vi "Version_2.0_Single_Column_Code.vi"() -> ()   [LabVIEW 2020] (continued)
                                n7833 = local read "Stop for End of \nExperiment \nand Data Writing"() -> (w8307:bool)
                                n7834 = call <vilib>:"Trim Whitespace.vi"("string"=w8319) -> ("trimmed string"=w8318:string)  [unwired: 1 in]
                                n7835 = Not(x=w8313) -> (.not. x?=w8311:bool)
                                n7836 = Equal?(x=w8318, y="/0`\u0003") -> (x = y?=w8316:bool)
                                n7837 = Or(x=w8311, y=w8310) -> (x .or. y?=w8309:bool)
                                n7838 = local read "Re-SEC"() -> (w8306:bool)
                                n7839 = Or(x=w8307, y=w8306) -> (x .or. y?=w8305:bool)
                                n7840 = Or(x=w8309, y=w8305) -> (x .or. y?=w8315:bool)
                                n7841 = Or(x=w8316, y=w8315) -> (x .or. y?=w8314:bool)
                                }
                                }
                                n7842 = Wait (ms)(milliseconds to wait=u32 100) -> ()  [unwired: 1 out]
                                }
                                n7843 = local write "Valve V2 Open"(FALSE ("Valve V2 Open")) -> ()
                                n7844 = local write "Valve V1 Open"(TRUE ("Valve V1 Open")) -> ()
                                n7845 = local write "External Valve \nOpen"(FALSE ("External Valve \nOpen")) -> ()
                                n7846 = local write "Volume being Injected \nin this process"(0.0) -> ()
                                }
                                frame #1 {
                                # "Keeps the on-chip valve V1, V2 and V3 closed,\nHalts also deposition onto the grid\nand waits for the 1st redeposit command. Once the command is issued\nit starts pumpoing and moves onto the next frame"
                                n7847 = stacked-sequence {
                                frame #0 {
                                n7848 = local write "Valve V1 Open"(FALSE ("Valve V1 Open")) -> ()
                                n7849 = local read "VISA Refnum in\nfor Pump"() -> (w8326:refnum<visa-resource-name>)
                                n7850 = local write "Valve V2 Open"(FALSE ("Valve V2 Open")) -> ()
                                n7851 = local write "Re-deposit Sample\nonto Grid"(FALSE ("Redeposit Sample\nonto Grid")) -> ()
                                n7852 = local write "Pause Data Collection"(TRUE ("Pause Data Collection")) -> ()
                                n7853 = call "HardStopCurrentProcess (SubVI).vi"("VISA Refnum in"=w8326) -> ()  [unwired: 11 in]
                                n7854 = local write "External Valve \nOpen"(FALSE ("External Valve \nOpen")) -> ()
                                }
                                frame #1 {
                                n7855 = while {
                                stop <- w8332 stop-if-true
                                n7856 = local read "Stop for End of \nExperiment \nand Data Writing"() -> (w8330:bool)
                                n7857 = local read "Re-SEC"() -> (w8331:bool)
                                n7858 = local read "Re-deposit Sample\nonto Grid"() -> (w8333:bool)
                                n7859 = Or(x=w8330, y=w8331) -> (x .or. y?=w8329:bool)
                                n7860 = Or(x=w8333, y=w8329) -> (x .or. y?=w8332:bool)
                                }
                                n7861 = local write "Discard fluid \nprior to 1st \ndeposition"(FALSE ("Discard fluid \nprior to 1st \ndeposition")) -> ()
                                n7862 = One Button Dialog(message="Do you want to deposit sample on another grid? If yes, turn on 'Re-deposit Sample onto Grid'. Else turn on Re-SEC to do SEC again or STOP to end the experiment") -> ()  [unwired: 1 in, 1 out]
                                }
                                frame #2 {
                                n7863 = local write "Valve V1 Open"(TRUE ("Valve V3 Open")) -> ()
                                }
                                frame #3 {
                                n7864 = local read "Re-deposit Sample\nonto Grid"() -> (w8335:bool)
                                n7865 = case shown="True" w8335 {
                                frame False {
                                n7866 = local write "Suction On/Off"(FALSE ("Suction On/Off")) -> ()
                                }
                                frame True {
                                n7867 = stacked-sequence {
                                frame #0 {
                                n7868 = local read "VISA Refnum in\nfor Pump"() -> (w8338:refnum<visa-resource-name>)
                                n7869 = call "AbsolutePlungerPosition (SubVI).vi"("VISA Refnum in"=w8338) -> ("Plunger Position"=w8337:i32)  [unwired: 10 in]
                                n7870 = local write "Position\nNow"(w8337) -> ()
                                }
                                frame #1 {
                                n7871 = local read "Buffer-B Pumping\nResolution"() -> (w8340:T2)
                                n7872 = case shown="\"Standard Pumping\", Default" w8340 {
                                tunnel: [w8341 w8352] -> w8339
                                frame "Standard Pumping", Default {
                                n7873 = local read "Buffer-B Volume \nto be  Pumped"() -> (w8344:dbl)
                                n7874 = local read "Volume of Syringe"() -> (w8347:dbl)
                                n7875 = local read "Initial Plunger Position"() -> (w8351:dbl)
                                n7876 = local read "Position\nNow"() -> (w8350:dbl)
                                n7877 = Subtract(x=w8351, y=w8350) -> (x-y=w8349:dbl)
                                n7878 = Absolute Value(x=w8349) -> (abs(x)=w8348:dbl)
                                n7879 = Multiply(x=w8348, y=w8347) -> (x*y=w8346:dbl)
                                n7880 = Divide(x=w8346, y=3000.0) -> (x/y=w8343:dbl)
                                n7881 = Subtract(x=w8343, y=w8344) -> (x-y=w8342:dbl)
                                n7882 = Absolute Value(x=w8342) -> (abs(x)=w8341:dbl)
                                }
                                frame "High Resolution Pumping" {
                                n7883 = local read "Buffer-C2 Volume \nto be Pumped"() -> (w8355:dbl)
                                n7884 = local read "Volume of Syringe"() -> (w8358:dbl)
                                n7885 = local read "Initial Plunger Position"() -> (w8362:dbl)
                                n7886 = local read "Position\nNow"() -> (w8361:dbl)
                                n7887 = Subtract(x=w8362, y=w8361) -> (x-y=w8360:dbl)
                                n7888 = Absolute Value(x=w8360) -> (abs(x)=w8359:dbl)
                                n7889 = Multiply(x=w8359, y=w8358) -> (x*y=w8357:dbl)
                                n7890 = Divide(x=w8357, y=24000.0) -> (x/y=w8354:dbl)
                                n7891 = Subtract(x=w8354, y=w8355) -> (x-y=w8353:dbl)
                                n7892 = Absolute Value(x=w8353) -> (abs(x)=w8352:dbl)
                                }
                                }
                                n7893 = local write "Buffer-C Volume\nleft to be Pumped"(w8339) -> ()
                                }
                                frame #2 {
                                n7894 = local read "Buffer-B Dispense\nFlow Rate (ul/min)"() -> (w8366:dbl)
                                n7895 = local read "Buffer-B Pumping\nResolution"() -> (w8365:T2)
                                n7896 = local read "VISA Refnum in\nfor Pump"() -> (w8368:refnum<visa-resource-name>)
                                n7897 = local read "Volume of Syringe"() -> (w8367:dbl)
                                n7898 = call "GoToAbsolutePosition(SubVI).vi"("Absolute Volume Position in Syringe (in ul)"=0.0, "Volume of Syringe"=w8367, "Resolution of Pumping"=w8365, "Flow Rate (ul/min)"=w8366, "VISA Refnum in"=w8368) -> ()  [unwired: 6 in, 1 out]
                                n7899 = local write "Suction On/Off"(FALSE ("Suction On/Off")) -> ()
                                }
                                }
                                }
                                }
                                }
                                frame #4 {
                                n7900 = local read "Stop for End of \nExperiment \nand Data Writing"() -> (w8371:bool)
                                n7901 = local read "Re-SEC"() -> (w8370:bool)
                                n7902 = Or(x=w8371, y=w8370) -> (x .or. y?=w8369:bool)
                                n7903 = case shown="True" w8369 {
                                frame False {
                                }
                                frame True {
                                n7904 = local read "VISA Refnum in\nfor Pump"() -> (w8372:refnum<visa-resource-name>)
                                n7905 = call "HardStopCurrentProcess (SubVI).vi"("VISA Refnum in"=w8372) -> ()  [unwired: 11 in]
                                }
                                }
                                }
                                }
                                }
                                frame #2 {
                                # "Keeps the on-chip valve V1, V2 Open and V3 closed"
                                n7906 = while {
                                stop <- w8378 stop-if-true
                                n7907 = local read "Suction On/Off"() -> (w8379:bool)
                                n7908 = case shown="True" w8379 {
                                frame False {
                                n7909 = local read "Initial Plunger Position"() -> (w8384:dbl)
                                n7910 = local read "Buffer-B Pumping\nResolution"() -> (w8385:T2)
                                n7911 = local read "VISA Refnum in\nfor Pump"() -> (w8386:refnum<visa-resource-name>)
                                n7912 = local read "Position\nNow"() -> (w8382:dbl)
                                n7913 = local read "Volume of Syringe"() -> (w8383:dbl)
                                n7914 = local write "Volume being Injected \nin this process"(0.0) -> ()
                                n7915 = local write "Pause Data Collection"(FALSE) -> ()
                                n7916 = while {
                                tunnel: w8386 -> [w8393]
                                tunnel: w8385 -> [w8392]
                                tunnel: w8384 -> [w8388]
                                tunnel: w8383 -> [w8391]
                                tunnel: w8382 -> [w8387]
                                stop <- w8389 stop-if-true
                                n7917 = stacked-sequence {
                                tunnel: w8393 -> [w8399 w8421 w8448]
                                tunnel: w8392 -> [w8398 w8420 _]
                                tunnel: w8388 -> [w8396 _ _]
                                tunnel: w8391 -> [w8395 w8418 _]
                                tunnel: [_ _ w8441] -> w8389
                                tunnel: w8387 -> [_ w8416 _]
                                frame #0 {
                                # "From here on 'True Volume being injected \nin this process' represents the true total \nvolume in this process"
                                n7918 = call "AbsolutePlungerPosition (SubVI).vi"("VISA Refnum in"=w8399) -> ("Plunger Position"=w8397:i32)  [unwired: 10 in]
                                n7919 = case shown="..\"Standard Pumping\"" w8398 {
                                tunnel: w8397 -> [w8407 w8415]
                                tunnel: w8396 -> [w8406 w8414]
                                tunnel: w8395 -> [w8403 w8411]
                                tunnel: [w8400 w8408] -> w8394
                                frame .."Standard Pumping" {
                                n7920 = Subtract(x=w8407, y=w8406) -> (x-y=w8405:dbl)
                                n7921 = Absolute Value(x=w8405) -> (abs(x)=w8404:dbl)
                                n7922 = Multiply(x=w8404, y=w8403) -> (x*y=w8402:dbl)
                                n7923 = Divide(x=w8402, y=3000.0) -> (x/y=w8400:dbl)
                                }
                                frame "High Resolution Pumping".. {
                                n7924 = Subtract(x=w8415, y=w8414) -> (x-y=w8413:dbl)
                                n7925 = Absolute Value(x=w8413) -> (abs(x)=w8412:dbl)
                                n7926 = Multiply(x=w8412, y=w8411) -> (x*y=w8410:dbl)
                                n7927 = Divide(x=w8410, y=24000.0) -> (x/y=w8408:dbl)
                                }
                                }
                                n7928 = local write "True Volume being \ninjected in this\nprocess"(w8394) -> ()
                                }
                                frame #1 {
                                # "From here on 'Volume being injected \nin this process' represents the volume \nin this sub process"
                                n7929 = call "AbsolutePlungerPosition (SubVI).vi"("VISA Refnum in"=w8421) -> ("Plunger Position"=w8419:i32)  [unwired: 10 in]
                                n7930 = case shown="\"High Resolution Pumping\".." w8420 {
                                tunnel: w8419 -> [w8429 w8437]
                                tunnel: w8416 -> [w8428 w8436]
                                tunnel: w8418 -> [w8425 w8433]
                                tunnel: [w8422 w8430] -> w8417
                                frame .."Standard Pumping" {
                                n7931 = Subtract(x=w8429, y=w8428) -> (x-y=w8427:dbl)
                                n7932 = Absolute Value(x=w8427) -> (abs(x)=w8426:dbl)
                                n7933 = Multiply(x=w8426, y=w8425) -> (x*y=w8424:dbl)
                                n7934 = Divide(x=w8424, y=3000.0) -> (x/y=w8422:dbl)
                                }
                                frame "High Resolution Pumping".. {
                                n7935 = Subtract(x=w8437, y=w8436) -> (x-y=w8435:dbl)
                                n7936 = Absolute Value(x=w8435) -> (abs(x)=w8434:dbl)
                                n7937 = Multiply(x=w8434, y=w8433) -> (x*y=w8432:dbl)
                                n7938 = Divide(x=w8432, y=24000.0) -> (x/y=w8430:dbl)
                                }
                                }
                                n7939 = local write "Volume being Injected \nin this process"(w8417) -> ()
                                }
                                frame #2 {
                                n7940 = local read "Stop for End of \nExperiment \nand Data Writing"() -> (w8440:bool)
                                n7941 = local read "Re-SEC"() -> (w8439:bool)
                                n7942 = local read "Suction On/Off"() -> (w8444:bool)
                                n7943 = call "AbsolutePlungerPositionStatus (SubVI).vi"("VISA Refnum in"=w8448) -> ("read buffer"=w8447:string)  [unwired: 10 in]
                                n7944 = call <vilib>:"Trim Whitespace.vi"("string"=w8447) -> ("trimmed string"=w8446:string)  [unwired: 1 in]
                                n7945 = Equal?(x=w8446, y="/0`\u0003") -> (x = y?=w8443:bool)
                                n7946 = Or(x=w8440, y=w8439) -> (x .or. y?=w8438:bool)
                                n7947 = Or(x=w8444, y=w8438) -> (x .or. y?=w8442:bool)
                                n7948 = Or(x=w8443, y=w8442) -> (x .or. y?=w8441:bool)
                                }
                                }
                                n7949 = Wait (ms)(milliseconds to wait=u32 100) -> ()  [unwired: 1 out]
                                }
                                }
                                frame True {
                                n7950 = stacked-sequence {
                                frame #0 {
                                n7951 = local write "Valve V1 Open"(FALSE ("Valve V3 Open")) -> ()
                                n7952 = local read "Suction Pressure\nfor EM-grid \nDeposition (mbar)"() -> (w8450:sgl)
                                n7953 = local read "VISA Refnum in\nfor Pump"() -> (w8453:refnum<visa-resource-name>)
                                n7954 = local write "Suction pressure \nfor grid deposition"(w8450) -> ()
                                n7955 = local write "Re-deposit Sample\nonto Grid"(FALSE ("Redeposit Sample\nonto Grid")) -> ()
                                n7956 = local write "Pause Data Collection"(TRUE ("Pause Data Collection")) -> ()
                                n7957 = call "HardStopCurrentProcess (SubVI).vi"("VISA Refnum in"=w8453) -> ()  [unwired: 11 in]
                                }
                                frame #1 {
                                n7958 = while {
                                stop <- w8456 stop-if-true
                                n7959 = local read "Stop for End of \nExperiment \nand Data Writing"() -> (w8457:bool)
                                n7960 = local read "Suction Pressure\nfor EM-grid \nDeposition (mbar)"() -> (w8454:sgl)
                                n7961 = call <vilib>:"fgt set pressure.vi"("pressure"=w8454, "pressureIndex"=u32 1) -> ()  [unwired: 9 in, 1 out]
                                n7962 = local read "Suction On/Off"() -> (w8459:bool)
                                n7963 = Not(x=w8459) -> (.not. x?=w8458:bool)
                                n7964 = Wait (ms)(milliseconds to wait=u32 100) -> ()  [unwired: 1 out]
                                n7965 = Or(x=w8458, y=w8457) -> (x .or. y?=w8456:bool)
                                }
                                }
                                frame #2 {
                                n7966 = for {
                                N: 2 -> [_]
                                n7967 = while {
                                stop <- w8469 stop-if-true
                                n7968 = local read "Stop for End of \nExperiment \nand Data Writing"() -> (w8465:bool)
                                n7969 = local read "Suction On/Off"() -> (w8467:bool)
                                n7970 = call <vilib>:"fgt set pressure.vi"("pressure"=sgl 0.0, "pressureIndex"=u32 1) -> ()  [unwired: 9 in, 1 out]
                                n7971 = Not(x=w8467) -> (.not. x?=w8466:bool)
                                n7972 = Wait (ms)(milliseconds to wait=u32 100) -> ()  [unwired: 1 out]
                                n7973 = Or(x=w8466, y=w8465) -> (x .or. y?=w8469:bool)
                                }
                                n7974 = Wait (ms)(milliseconds to wait=u32 400) -> ()  [unwired: 1 out]
                                }
                                }
                                frame #3 {
                                n7975 = local read "Automatic purging \nof capillary after \ngrid deposition"() -> (w8470:bool)
                                n7976 = case shown="True" w8470 {
                                frame False {
                                }
                                frame True {
                                n7977 = stacked-sequence {
                                frame #0 {
                                n7978 = local read "VISA Refnum in\nfor Pump"() -> (w8472:refnum<visa-resource-name>)
                                n7979 = call "AbsolutePlungerPosition (SubVI).vi"("VISA Refnum in"=w8472) -> ("Plunger Position"=w8471:i32)  [unwired: 10 in]
                                n7980 = local write "Position\nNow"(w8471) -> ()
                                }
                                frame #1 {
                                n7981 = local read "Buffer-B Pumping\nResolution"() -> (w8474:T2)
                                n7982 = case shown="\"Standard Pumping\", Default" w8474 {
                                tunnel: [w8475 w8486] -> w8473
                                frame "Standard Pumping", Default {
                                n7983 = local read "Buffer-B Volume \nto be  Pumped"() -> (w8478:dbl)
                                n7984 = local read "Volume of Syringe"() -> (w8481:dbl)
                                n7985 = local read "Initial Plunger Position"() -> (w8485:dbl)
                                n7986 = local read "Position\nNow"() -> (w8484:dbl)
                                n7987 = Subtract(x=w8485, y=w8484) -> (x-y=w8483:dbl)
                                n7988 = Absolute Value(x=w8483) -> (abs(x)=w8482:dbl)
                                n7989 = Multiply(x=w8482, y=w8481) -> (x*y=w8480:dbl)
                                n7990 = Divide(x=w8480, y=3000.0) -> (x/y=w8477:dbl)
                                n7991 = Subtract(x=w8477, y=w8478) -> (x-y=w8476:dbl)
                                n7992 = Absolute Value(x=w8476) -> (abs(x)=w8475:dbl)
                                }
                                frame "High Resolution Pumping" {
                                n7993 = local read "Buffer-C2 Volume \nto be Pumped"() -> (w8489:dbl)
                                n7994 = local read "Volume of Syringe"() -> (w8492:dbl)
                                n7995 = local read "Initial Plunger Position"() -> (w8496:dbl)
                                n7996 = local read "Position\nNow"() -> (w8495:dbl)
                                n7997 = Subtract(x=w8496, y=w8495) -> (x-y=w8494:dbl)
                                n7998 = Absolute Value(x=w8494) -> (abs(x)=w8493:dbl)
                                n7999 = Multiply(x=w8493, y=w8492) -> (x*y=w8491:dbl)
                                n8000 = Divide(x=w8491, y=24000.0) -> (x/y=w8488:dbl)
                                n8001 = Subtract(x=w8488, y=w8489) -> (x-y=w8487:dbl)
                                n8002 = Absolute Value(x=w8487) -> (abs(x)=w8486:dbl)
                                }
                                }
                                n8003 = local write "Buffer-C Volume\nleft to be Pumped"(w8473) -> ()
                                }
                                frame #2 {
                                n8004 = local read "Buffer-B Dispense\nFlow Rate (ul/min)"() -> (w8500:dbl)
                                n8005 = local read "Buffer-B Pumping\nResolution"() -> (w8499:T2)
                                n8006 = local read "VISA Refnum in\nfor Pump"() -> (w8502:refnum<visa-resource-name>)
                                n8007 = local read "Volume of Syringe"() -> (w8501:dbl)
                                n8008 = call "GoToAbsolutePosition(SubVI).vi"("Absolute Volume Position in Syringe (in ul)"=0.0, "Volume of Syringe"=w8501, "Resolution of Pumping"=w8499, "Flow Rate (ul/min)"=w8500, "VISA Refnum in"=w8502) -> ()  [unwired: 6 in, 1 out]
                                n8009 = local write "Valve V1 Open"(TRUE ("Valve V3 Open")) -> ()
                                }
                                frame #3 {
                                n8010 = local read "Initial Plunger Position"() -> (w8507:dbl)
                                n8011 = local read "Buffer-B Pumping\nResolution"() -> (w8508:T2)
                                n8012 = local read "VISA Refnum in\nfor Pump"() -> (w8509:refnum<visa-resource-name>)
                                n8013 = local read "Position\nNow"() -> (w8505:dbl)
                                n8014 = local read "Volume of Syringe"() -> (w8506:dbl)
                                n8015 = local write "Volume being Injected \nin this process"(0.0) -> ()
                                n8016 = local write "Pause Data Collection"(FALSE) -> ()
                                n8017 = while {
                                tunnel: w8509 -> [w8516]
                                tunnel: w8508 -> [w8515]
                                tunnel: w8507 -> [w8511]
                                tunnel: w8506 -> [w8514]
                                tunnel: w8505 -> [w8510]
                                stop <- w8512 stop-if-true
                                n8018 = stacked-sequence {
                                tunnel: w8516 -> [w8522 w8544 w8573]
                                tunnel: w8515 -> [w8521 w8543 _]
                                tunnel: w8511 -> [w8519 _ _]
                                tunnel: w8514 -> [w8518 w8541 _]
                                tunnel: [_ _ w8567] -> w8512
                                tunnel: w8510 -> [_ w8539 _]
                                frame #0 {
                                # "From here on 'True Volume being injected \nin this process' represents the true total \nvolume in this process"
                                n8019 = call "AbsolutePlungerPosition (SubVI).vi"("VISA Refnum in"=w8522) -> ("Plunger Position"=w8520:i32)  [unwired: 10 in]
                                n8020 = case shown="..\"Standard Pumping\"" w8521 {
                                tunnel: w8520 -> [w8530 w8538]
                                tunnel: w8519 -> [w8529 w8537]
                                tunnel: w8518 -> [w8526 w8534]
                                tunnel: [w8523 w8531] -> w8517
                                frame .."Standard Pumping" {
                                n8021 = Subtract(x=w8530, y=w8529) -> (x-y=w8528:dbl)
                                n8022 = Absolute Value(x=w8528) -> (abs(x)=w8527:dbl)
                                n8023 = Multiply(x=w8527, y=w8526) -> (x*y=w8525:dbl)
                                n8024 = Divide(x=w8525, y=3000.0) -> (x/y=w8523:dbl)
                                }
                                frame "High Resolution Pumping".. {
                                n8025 = Subtract(x=w8538, y=w8537) -> (x-y=w8536:dbl)
                                n8026 = Absolute Value(x=w8536) -> (abs(x)=w8535:dbl)
                                n8027 = Multiply(x=w8535, y=w8534) -> (x*y=w8533:dbl)
                                n8028 = Divide(x=w8533, y=24000.0) -> (x/y=w8531:dbl)
                                }
                                }
                                n8029 = local write "True Volume being \ninjected in this\nprocess"(w8517) -> ()
                                }
                                frame #1 {
                                # "From here on 'Volume being injected \nin this process' represents the volume \nin this sub process"
                                n8030 = call "AbsolutePlungerPosition (SubVI).vi"("VISA Refnum in"=w8544) -> ("Plunger Position"=w8542:i32)  [unwired: 10 in]
                                n8031 = case shown="\"High Resolution Pumping\".." w8543 {
                                tunnel: w8542 -> [w8552 w8560]
                                tunnel: w8539 -> [w8551 w8559]
                                tunnel: w8541 -> [w8548 w8556]
                                tunnel: [w8545 w8553] -> w8540
                                frame .."Standard Pumping" {
                                n8032 = Subtract(x=w8552, y=w8551) -> (x-y=w8550:dbl)
                                n8033 = Absolute Value(x=w8550) -> (abs(x)=w8549:dbl)
                                n8034 = Multiply(x=w8549, y=w8548) -> (x*y=w8547:dbl)
                                n8035 = Divide(x=w8547, y=3000.0) -> (x/y=w8545:dbl)
                                }
                                frame "High Resolution Pumping".. {
                                n8036 = Subtract(x=w8560, y=w8559) -> (x-y=w8558:dbl)
                                n8037 = Absolute Value(x=w8558) -> (abs(x)=w8557:dbl)
                                n8038 = Multiply(x=w8557, y=w8556) -> (x*y=w8555:dbl)
                                n8039 = Divide(x=w8555, y=24000.0) -> (x/y=w8553:dbl)
                                }
                                }
                                n8040 = local write "Volume being Injected \nin this process"(w8540) -> ()
                                }
                                frame #2 {
                                n8041 = local read "Capillary purge \nvolume after every\ngrid plunging"() -> (w8562:dbl)
                                n8042 = local read "Stop for End of \nExperiment \nand Data Writing"() -> (w8566:bool)
                                n8043 = local read "Volume being Injected \nin this process"() -> (w8563:dbl)
                                n8044 = local read "Re-SEC"() -> (w8565:bool)
                                n8045 = call "AbsolutePlungerPositionStatus (SubVI).vi"("VISA Refnum in"=w8573) -> ("read buffer"=w8572:string)  [unwired: 10 in]
                                n8046 = call <vilib>:"Trim Whitespace.vi"("string"=w8572) -> ("trimmed string"=w8571:string)  [unwired: 1 in]
                                n8047 = Greater Or Equal?(x=w8563, y=w8562) -> (x >= y?=w8561:bool)
                                n8048 = Equal?(x=w8571, y="/0`\u0003") -> (x = y?=w8569:bool)
                                n8049 = Or(x=w8566, y=w8565) -> (x .or. y?=w8564:bool)
                                n8050 = Or(x=w8561, y=w8564) -> (x .or. y?=w8568:bool)
                                n8051 = Or(x=w8569, y=w8568) -> (x .or. y?=w8567:bool)
                                }
                                }
                                n8052 = Wait (ms)(milliseconds to wait=u32 100) -> ()  [unwired: 1 out]
                                }
                                }
                                frame #4 {
                                n8053 = local read "VISA Refnum in\nfor Pump"() -> (w8574:refnum<visa-resource-name>)
                                n8054 = call "HardStopCurrentProcess (SubVI).vi"("VISA Refnum in"=w8574) -> ()  [unwired: 11 in]
                                }
                                }
                                }
                                }
                                }
                                frame #4 {
                                n8055 = local write "Valve V1 Open"(FALSE ("Valve V3 Open")) -> ()
                                }
                                frame #5 {
                                n8056 = while {
                                stop <- w8580 stop-if-true
                                n8057 = local read "Stop for End of \nExperiment \nand Data Writing"() -> (w8578:bool)
                                n8058 = local read "Re-deposit Sample\nonto Grid"() -> (w8581:bool)
                                n8059 = local read "Re-SEC"() -> (w8579:bool)
                                n8060 = Or(x=w8578, y=w8579) -> (x .or. y?=w8577:bool)
                                n8061 = Or(x=w8581, y=w8577) -> (x .or. y?=w8580:bool)
                                }
                                n8062 = One Button Dialog(message="Do you want to deposit sample on another grid? If yes, turn on 'Re-deposit Sample onto Grid'. Else turn on Re-SEC to do SEC again or STOP to end the experiment") -> ()  [unwired: 1 in, 1 out]
                                }
                                frame #6 {
                                n8063 = local write "Valve V1 Open"(TRUE ("Valve V3 Open")) -> ()
                                }
                                frame #7 {
                                n8064 = local read "Re-deposit Sample\nonto Grid"() -> (w8583:bool)
                                n8065 = case shown="True" w8583 {
                                frame False {
                                n8066 = local write "Suction On/Off"(FALSE ("Suction On/Off")) -> ()
                                }
                                frame True {
                                n8067 = stacked-sequence {
                                frame #0 {
                                n8068 = local read "VISA Refnum in\nfor Pump"() -> (w8586:refnum<visa-resource-name>)
                                n8069 = call "AbsolutePlungerPosition (SubVI).vi"("VISA Refnum in"=w8586) -> ("Plunger Position"=w8585:i32)  [unwired: 10 in]
                                n8070 = local write "Position\nNow"(w8585) -> ()
                                }
                                frame #1 {
                                n8071 = local read "Buffer-B Pumping\nResolution"() -> (w8588:T2)
                                n8072 = case shown="\"Standard Pumping\", Default" w8588 {
                                tunnel: [w8589 w8600] -> w8587
                                frame "Standard Pumping", Default {
                                n8073 = local read "Buffer-B Volume \nto be  Pumped"() -> (w8592:dbl)
                                n8074 = local read "Volume of Syringe"() -> (w8595:dbl)
                                n8075 = local read "Initial Plunger Position"() -> (w8599:dbl)
                                n8076 = local read "Position\nNow"() -> (w8598:dbl)
                                n8077 = Subtract(x=w8599, y=w8598) -> (x-y=w8597:dbl)
                                n8078 = Absolute Value(x=w8597) -> (abs(x)=w8596:dbl)
                                n8079 = Multiply(x=w8596, y=w8595) -> (x*y=w8594:dbl)
                                n8080 = Divide(x=w8594, y=3000.0) -> (x/y=w8591:dbl)
                                n8081 = Subtract(x=w8591, y=w8592) -> (x-y=w8590:dbl)
                                n8082 = Absolute Value(x=w8590) -> (abs(x)=w8589:dbl)
                                }
                                frame "High Resolution Pumping" {
                                n8083 = local read "Buffer-C2 Volume \nto be Pumped"() -> (w8603:dbl)
                                n8084 = local read "Volume of Syringe"() -> (w8606:dbl)
                                n8085 = local read "Initial Plunger Position"() -> (w8610:dbl)
                                n8086 = local read "Position\nNow"() -> (w8609:dbl)
                                n8087 = Subtract(x=w8610, y=w8609) -> (x-y=w8608:dbl)
                                n8088 = Absolute Value(x=w8608) -> (abs(x)=w8607:dbl)
                                n8089 = Multiply(x=w8607, y=w8606) -> (x*y=w8605:dbl)
                                n8090 = Divide(x=w8605, y=24000.0) -> (x/y=w8602:dbl)
                                n8091 = Subtract(x=w8602, y=w8603) -> (x-y=w8601:dbl)
                                n8092 = Absolute Value(x=w8601) -> (abs(x)=w8600:dbl)
                                }
                                }
                                n8093 = local write "Buffer-C Volume\nleft to be Pumped"(w8587) -> ()
                                }
                                frame #2 {
                                n8094 = local read "Buffer-B Dispense\nFlow Rate (ul/min)"() -> (w8614:dbl)
                                n8095 = local read "Buffer-B Pumping\nResolution"() -> (w8613:T2)
                                n8096 = local read "VISA Refnum in\nfor Pump"() -> (w8616:refnum<visa-resource-name>)
                                n8097 = local read "Volume of Syringe"() -> (w8615:dbl)
                                n8098 = call "GoToAbsolutePosition(SubVI).vi"("Absolute Volume Position in Syringe (in ul)"=0.0, "Volume of Syringe"=w8615, "Resolution of Pumping"=w8613, "Flow Rate (ul/min)"=w8614, "VISA Refnum in"=w8616) -> ()  [unwired: 6 in, 1 out]
                                n8099 = local write "Suction On/Off"(FALSE ("Suction On/Off")) -> ()
                                }
                                }
                                }
                                }
                                }
                                frame #8 {
                                n8100 = local read "Stop for End of \nExperiment \nand Data Writing"() -> (w8618:bool)
                                n8101 = local read "Re-SEC"() -> (w8619:bool)
                                n8102 = Or(x=w8618, y=w8619) -> (x .or. y?=w8617:bool)
                                n8103 = case shown="True" w8617 {
                                frame False {
                                }
                                frame True {
                                n8104 = local read "VISA Refnum in\nfor Pump"() -> (w8620:refnum<visa-resource-name>)
                                n8105 = call "HardStopCurrentProcess (SubVI).vi"("VISA Refnum in"=w8620) -> ()  [unwired: 11 in]
                                }
                                }
                                }
                                }
                                }
                                }
                                n8106 = local read "Stop for End of \nExperiment \nand Data Writing"() -> (w8374:bool)
                                n8107 = local read "Divert Sample \nonto Grid"() -> (w8377:bool)
                                n8108 = local read "Re-SEC"() -> (w8375:bool)
                                n8109 = Not(x=w8377) -> (.not. x?=w8376:bool)
                                n8110 = Or(x=w8374, y=w8375) -> (x .or. y?=w8373:bool)
                                n8111 = Or(x=w8376, y=w8373) -> (x .or. y?=w8378:bool)
                                }
                                }
                                }
                                n8112 = local write "Discard fluid \nprior to 1st \ndeposition"(TRUE ("Discard fluid \nprior to 1st \ndeposition")) -> ()
                                }
                                }
                              }
                              frame #9 {
                                n8113 = local write "Pause Data Collection"(TRUE ("Pause Data Collection")) -> ()
                                n8114 = Wait (ms)(milliseconds to wait=u32 500) -> ()  [unwired: 1 out]
                              }
                              frame #10 {
                                n8115 = local write "Volume being Injected \nin this process"(0.0 ("Volume being Injected \nin this process")) -> ()
                                n8116 = local write "Affinity Elution On"(FALSE ("Affinity Elution On")) -> ()
                                n8117 = local write "Start the Process"(FALSE ("Start the Process")) -> ()
                              }
                            }
                          }
                        }
                        n8118 = local write "Washing Column-1"(FALSE ("Sample pumping \ninto Column-1")) -> ()
                        n8119 = local write "Elution of Column-1"(TRUE ("Washing Column-1")) -> ()
                        n8120 = local write "Affinity Elution On"(TRUE ("Affinity Elution On")) -> ()
                      }
                    }
                  }
                }
              }
              frame True {
                n8121 = local write "Pause Data Collection"(FALSE ("Pause Data Collection")) -> ()
              }
            }
          }
          frame "Inject Buffer A2, Column 1 with 4 SOD Valves" {
            n8122 = local read "Stopper that ends \nthe main loops"() -> (w8627:bool)
            n8123 = case shown="False" w8627 {
              frame False {
                n8124 = local read "Start the Process"() -> (w8628:bool)
                n8125 = case shown="True" w8628 {
                  frame False {
                    n8126 = local read "Stopper that ends \nthe main loops"() -> (w8630:bool)
                    n8127 = local read "Start the Process"() -> (w8629:bool)
                    n8128 = Or(x=w8630, y=w8629) -> (x .or. y?=w8631:bool)
                    n8129 = case shown="False" w8631 {
                      frame False {
                        n8130 = while {
                          stop <- w8634 stop-if-true
                          n8131 = local read "Stop for End of \nExperiment \nand Data Writing"() -> (w8633:bool)
                          n8132 = local read "Stopper that ends \nthe main loops"() -> (w8636:bool)
                          n8133 = local read "Start the Process"() -> (w8635:bool)
                          n8134 = Wait (ms)(milliseconds to wait=u32 10) -> ()  [unwired: 1 out]
                          n8135 = Or(x=w8636, y=w8635) -> (x .or. y?=w8634:bool)
                          n8136 = local write "Stopper that ends \nthe main loops"(w8633) -> ()
                        }
                        n8137 = One Button Dialog(message="Please Select the Process and Press 'Start the Process' Button") -> ()  [unwired: 1 in, 1 out]
                      }
                      frame True {
                      }
                    }
                  }
                  frame True {
                    n8138 = stacked-sequence {
                      frame #0 {
                        n8139 = local read "Buffer-A2 Volume \nto be Pumped"() -> (w8641:dbl)
                        n8140 = local read "Apparent Volume\nof Syringe"() -> (w8640:dbl)
                        n8141 = Quotient & Remainder(x=w8641, y=w8640) -> (x-y*floor(x/y)=w8638:dbl, floor(x/y)=w8639:dbl)
                        n8142 = for {
                          N: w8639 -> [_]
                          n8143 = stacked-sequence {
                            frame #0 {
                              # "Switch to Port-4"
                              # "Port-4 of pump is connected to Buffer-A"
                              n8144 = local read "VISA Refnum in\nfor Pump"() -> (w8643:refnum<visa-resource-name>)
                              n8145 = local read "Port for \nA2-Wash"() -> (w8642:string)
                              n8146 = call "PortChanger (SubVI).vi"("Port Number"=w8642, "VISA Refnum in"=w8643) -> ()  [unwired: 10 in]
                            }
                            frame #1 {
                              n8147 = local read "VISA Refnum in\nfor Pump"() -> (w8644:refnum<visa-resource-name>)
                              n8148 = call "ProcessCompletionWaiter (SubVI).vi"("VISA Refnum in"=w8644) -> ()  [unwired: 11 in]
                            }
                            frame #2 {
                              n8149 = local read "Buffer-A2 PickUp \nFlow Rate (ul/min)"() -> (w8647:dbl)
                              n8150 = local read "Buffer-A2 Pumping\nResolution"() -> (w8646:T2)
                              n8151 = local read "VISA Refnum in\nfor Pump"() -> (w8649:refnum<visa-resource-name>)
                              n8152 = local read "Apparent Volume\nof Syringe"() -> (w8645:dbl)
                              n8153 = local read "Volume of Syringe"() -> (w8648:dbl)
                              n8154 = call "RPickUp(SubVI).vi"("Volume to be picked up"=w8645, "Volume of Syringe"=w8648, "Resolution of PickUP"=w8646, "PickUp Flow Rate (ul/min)"=w8647, "VISA Refnum in"=w8649) -> ()  [unwired: 6 in, 1 out]
                            }
                            frame #3 {
                              n8155 = local read "Stopper that ends \nthe main loops"() -> (w8650:bool)
                              n8156 = local read "VISA Refnum in\nfor Pump"() -> (w8651:refnum<visa-resource-name>)
                              n8157 = case shown="True" w8650 {
                                frame False {
                                }
                                frame True {
                                n8158 = local read "VISA Refnum in\nfor Pump"() -> (w8652:refnum<visa-resource-name>)
                                n8159 = call "HardStopCurrentProcess (SubVI).vi"("VISA Refnum in"=w8652) -> ()  [unwired: 11 in]
                                }
                              }
                              n8160 = call "ProcessCompletionWaiter (SubVI).vi"("VISA Refnum in"=w8651) -> ()  [unwired: 11 in]
                            }
                            frame #4 {
                              # "Reads the initial Plunger Position for computing the volume dispensed"
                              n8161 = local read "VISA Refnum in\nfor Pump"() -> (w8654:refnum<visa-resource-name>)
                              n8162 = call "AbsolutePlungerPosition (SubVI).vi"("VISA Refnum in"=w8654) -> ("Plunger Position"=w8653:i32)  [unwired: 10 in]
                              n8163 = local write "Initial Plunger Position"(w8653) -> ()
                            }
                            frame #5 {
                              # "Switch to Port-2"
                              # "Port-2 of the pump is conncted to column-1 of chip"
                              n8164 = local read "VISA Refnum in\nfor Pump"() -> (w8656:refnum<visa-resource-name>)
                              n8165 = call "PortChanger (SubVI).vi"("Port Number"="2", "VISA Refnum in"=w8656) -> ()  [unwired: 10 in]
                            }
                            frame #6 {
                              n8166 = local read "Stopper that ends \nthe main loops"() -> (w8657:bool)
                              n8167 = local read "VISA Refnum in\nfor Pump"() -> (w8658:refnum<visa-resource-name>)
                              n8168 = case shown="True" w8657 {
                                frame False {
                                }
                                frame True {
                                n8169 = local read "VISA Refnum in\nfor Pump"() -> (w8659:refnum<visa-resource-name>)
                                n8170 = call "HardStopCurrentProcess (SubVI).vi"("VISA Refnum in"=w8659) -> ()  [unwired: 11 in]
                                }
                              }
                              n8171 = call "ProcessCompletionWaiter (SubVI).vi"("VISA Refnum in"=w8658) -> ()  [unwired: 11 in]
                            }
                            frame #7 {
                              # "Keeps the AMF valve after column-1 open and valve after column-2 closed"
                              n8172 = local read "Buffer-A2 Dispense\nFlow Rate (ul/min)"() -> (w8672:dbl)
                              n8173 = local read "Buffer-A2 Pumping\nResolution"() -> (w8671:T2)
                              n8174 = local read "VISA Refnum in\nfor Pump"() -> (w8674:refnum<visa-resource-name>)
                              n8175 = local write "Pause Data Collection"(FALSE ("Pause Data Collection")) -> ()
                              n8176 = local write "Valve V3 Open"(FALSE ("Valve V3 Open")) -> ()
                              n8177 = local write "Valve V4 Open"(FALSE ("Valve V4 Open")) -> ()
                              n8178 = local write "Valve V1 Open"(TRUE ("Valve V1 Open")) -> ()
                              n8179 = local write "Valve V2 Open"(TRUE ("Valve V2 Open")) -> ()
                              n8180 = local read "Volume of Syringe"() -> (w8673:dbl)
                              n8181 = call "GoToAbsolutePosition(SubVI).vi"("Absolute Volume Position in Syringe (in ul)"=0.0 ("Volume to be Dispensed"), "Volume of Syringe"=w8673, "Resolution of Pumping"=w8671, "Flow Rate (ul/min)"=w8672, "VISA Refnum in"=w8674) -> ()  [unwired: 6 in, 1 out]
                              n8182 = local write "External Valve \nOpen"(TRUE ("External Valve \nOpen")) -> ()
                              n8183 = local write "Valve V8 Open"(FALSE ("Valve V8 Open")) -> ()
                              n8184 = local write "Valve V5 Open"(FALSE ("Valve V5 Open")) -> ()
                              n8185 = local write "Valve V6 Open"(FALSE ("Valve V6 Open")) -> ()
                              n8186 = local write "Valve V7 Open"(FALSE ("Valve V7 Open")) -> ()
                            }
                            frame #8 {
                              n8187 = local read "Initial Plunger Position"() -> (w8677:dbl)
                              n8188 = local read "Buffer-A2 Pumping\nResolution"() -> (w8676:T2)
                              n8189 = local read "VISA Refnum in\nfor Pump"() -> (w8678:refnum<visa-resource-name>)
                              n8190 = local read "Volume of Syringe"() -> (w8675:dbl)
                              n8191 = while {
                                tunnel: w8677 -> [w8684]
                                tunnel: w8678 -> [w8683]
                                tunnel: w8676 -> [w8682]
                                tunnel: w8675 -> [w8681]
                                stop <- w8679 stop-if-true
                                n8192 = Wait (ms)(milliseconds to wait=u32 100) -> ()  [unwired: 1 out]
                                n8193 = stacked-sequence {
                                tunnel: w8684 -> [w8690 _]
                                tunnel: w8683 -> [w8689 w8710]
                                tunnel: w8682 -> [w8688 _]
                                tunnel: w8681 -> [w8687 _]
                                tunnel: [_ w8707] -> w8679
                                frame #0 {
                                n8194 = call "AbsolutePlungerPosition (SubVI).vi"("VISA Refnum in"=w8689) -> ("Plunger Position"=w8686:i32)  [unwired: 10 in]
                                n8195 = case shown="\"Standard Pumping\", Default" w8688 {
                                tunnel: w8690 -> [w8695 w8704]
                                tunnel: w8686 -> [w8696 w8703]
                                tunnel: [w8694 w8701] -> w8685
                                tunnel: w8687 -> [w8693 w8702]
                                frame "Standard Pumping", Default {
                                n8196 = Subtract(x=w8695, y=w8696) -> (x-y=w8692:dbl)
                                n8197 = Absolute Value(x=w8692) -> (abs(x)=w8691:dbl)
                                n8198 = Multiply(x=w8691, y=w8693) -> (x*y=w8698:dbl)
                                n8199 = Divide(x=w8698, y=3000.0) -> (x/y=w8694:dbl)
                                }
                                frame "High Resolution Pumping" {
                                n8200 = Subtract(x=w8704, y=w8703) -> (x-y=w8700:dbl)
                                n8201 = Absolute Value(x=w8700) -> (abs(x)=w8699:dbl)
                                n8202 = Multiply(x=w8699, y=w8702) -> (x*y=w8706:dbl)
                                n8203 = Divide(x=w8706, y=24000.0) -> (x/y=w8701:dbl)
                                }
                                }
                                n8204 = local write "Volume being Injected \nin this process"(w8685) -> ()
                                }
                                frame #1 {
                                n8205 = local read "Stop for End of \nExperiment \nand Data Writing"() -> (w8709:bool)
                                n8206 = call "LSPOneStatus (SubVI).vi"("VISA Refnum in"=w8710) -> ("read buffer"=w8712:string)  [unwired: 10 in]
                                n8207 = call <vilib>:"Trim Whitespace.vi"("string"=w8712) -> ("trimmed string"=w8711:string)  [unwired: 1 in]
                                n8208 = Equal?(x=w8711, y="/0`\u0003") -> (x = y?=w8708:bool)
                                n8209 = Or(x=w8708, y=w8709) -> (x .or. y?=w8707:bool)
                                }
                                }
                              }
                            }
                            frame #9 {
                              n8210 = local read "Stop for End of \nExperiment \nand Data Writing"() -> (w8714:bool)
                              n8211 = local write "Pause Data Collection"(TRUE ("Pause Data Collection")) -> ()
                              n8212 = local write "Valve V3 Open"(FALSE ("Valve V3 Open")) -> ()
                              n8213 = local write "Valve V2 Open"(FALSE ("Valve V2 Open")) -> ()
                              n8214 = local write "Valve V4 Open"(FALSE ("Valve V4 Open")) -> ()
                              n8215 = local write "Valve V1 Open"(FALSE ("Valve V1 Open")) -> ()
                              n8216 = Wait (ms)(milliseconds to wait=u32 500) -> ()  [unwired: 1 out]
                              n8217 = case shown="True" w8714 {
                                frame False {
                                }
                                frame True {
                                n8218 = local read "VISA Refnum in\nfor Pump"() -> (w8724:refnum<visa-resource-name>)
                                n8219 = call "HardStopCurrentProcess (SubVI).vi"("VISA Refnum in"=w8724) -> ()  [unwired: 11 in]
                                }
                              }
                              n8220 = local write "Valve V5 Open"(FALSE ("Valve V5 Open")) -> ()
                              n8221 = local write "Valve V6 Open"(FALSE ("Valve V6 Open")) -> ()
                              n8222 = local write "Valve V7 Open"(FALSE ("Valve V7 Open")) -> ()
                            }
                            frame #10 {
                              n8223 = local write "Volume being Injected \nin this process"(0.0 ("Volume being Injected \nin this process")) -> ()
                            }
                          }
                        }
                        n8224 = local write "Reminder of the \nVolume to be \nPumped"(w8638) -> ()
                      }
                      frame #1 {
                        n8225 = stacked-sequence {
                          frame #0 {
                            # "Switch to Port-4"
                            # "Port-4 of pump is connected to Buffer-A"
                            n8226 = local read "VISA Refnum in\nfor Pump"() -> (w8727:refnum<visa-resource-name>)
                            n8227 = local read "Port for \nA2-Wash"() -> (w8726:string)
                            n8228 = call "PortChanger (SubVI).vi"("Port Number"=w8726, "VISA Refnum in"=w8727) -> ()  [unwired: 10 in]
                          }
                          frame #1 {
                            n8229 = local read "VISA Refnum in\nfor Pump"() -> (w8728:refnum<visa-resource-name>)
                            n8230 = call "ProcessCompletionWaiter (SubVI).vi"("VISA Refnum in"=w8728) -> ()  [unwired: 11 in]
                          }
                          frame #2 {
                            n8231 = local read "Buffer-A2 PickUp \nFlow Rate (ul/min)"() -> (w8731:dbl)
                            n8232 = local read "Buffer-A2 Pumping\nResolution"() -> (w8730:T2)
                            n8233 = local read "VISA Refnum in\nfor Pump"() -> (w8733:refnum<visa-resource-name>)
                            n8234 = local read "Reminder of the \nVolume to be \nPumped"() -> (w8729:dbl)
                            n8235 = local read "Volume of Syringe"() -> (w8732:dbl)
                            n8236 = call "RPickUp(SubVI).vi"("Volume to be picked up"=w8729, "Volume of Syringe"=w8732, "Resolution of PickUP"=w8730, "PickUp Flow Rate (ul/min)"=w8731, "VISA Refnum in"=w8733) -> ()  [unwired: 6 in, 1 out]
                          }
                          frame #3 {
                            n8237 = local read "Stopper that ends \nthe main loops"() -> (w8734:bool)
                            n8238 = local read "VISA Refnum in\nfor Pump"() -> (w8735:refnum<visa-resource-name>)
                            n8239 = case shown="True" w8734 {
                              frame False {
                              }
                              frame True {
                                n8240 = local read "VISA Refnum in\nfor Pump"() -> (w8736:refnum<visa-resource-name>)
                                n8241 = call "HardStopCurrentProcess (SubVI).vi"("VISA Refnum in"=w8736) -> ()  [unwired: 11 in]
                              }
                            }
                            n8242 = call "ProcessCompletionWaiter (SubVI).vi"("VISA Refnum in"=w8735) -> ()  [unwired: 11 in]
                          }
                          frame #4 {
                            # "Reads the initial Plunger Position for computing the volume dispensed"
                            n8243 = local read "VISA Refnum in\nfor Pump"() -> (w8738:refnum<visa-resource-name>)
                            n8244 = call "AbsolutePlungerPosition (SubVI).vi"("VISA Refnum in"=w8738) -> ("Plunger Position"=w8737:i32)  [unwired: 10 in]
                            n8245 = local write "Initial Plunger Position"(w8737) -> ()
                          }
                          frame #5 {
                            # "Switch to Port-2"
                            # "Port-2 of the pump is conncted to column-1 of chip"
                            n8246 = local read "VISA Refnum in\nfor Pump"() -> (w8740:refnum<visa-resource-name>)
                            n8247 = call "PortChanger (SubVI).vi"("Port Number"="2", "VISA Refnum in"=w8740) -> ()  [unwired: 10 in]
                          }
                          frame #6 {
                            n8248 = local read "Stopper that ends \nthe main loops"() -> (w8741:bool)
                            n8249 = local read "VISA Refnum in\nfor Pump"() -> (w8742:refnum<visa-resource-name>)
                            n8250 = case shown="True" w8741 {
                              frame False {
                              }
                              frame True {
                                n8251 = local read "VISA Refnum in\nfor Pump"() -> (w8743:refnum<visa-resource-name>)
                                n8252 = call "HardStopCurrentProcess (SubVI).vi"("VISA Refnum in"=w8743) -> ()  [unwired: 11 in]
                              }
                            }
                            n8253 = call "ProcessCompletionWaiter (SubVI).vi"("VISA Refnum in"=w8742) -> ()  [unwired: 11 in]
                          }
                          frame #7 {
                            # "Keeps the AMF valve after column-1 open and valve after column-2 closed"
                            n8254 = local read "Buffer-A2 Dispense\nFlow Rate (ul/min)"() -> (w8756:dbl)
                            n8255 = local read "Buffer-A2 Pumping\nResolution"() -> (w8755:T2)
                            n8256 = local read "VISA Refnum in\nfor Pump"() -> (w8758:refnum<visa-resource-name>)
                            n8257 = local write "Pause Data Collection"(FALSE ("Pause Data Collection")) -> ()
                            n8258 = local write "Valve V3 Open"(FALSE ("Valve V3 Open")) -> ()
                            n8259 = local write "Valve V4 Open"(FALSE ("Valve V4 Open")) -> ()
                            n8260 = local write "Valve V1 Open"(TRUE ("Valve V1 Open")) -> ()
                            n8261 = local write "Valve V2 Open"(TRUE ("Valve V2 Open")) -> ()
                            n8262 = local read "Volume of Syringe"() -> (w8757:dbl)
                            n8263 = call "GoToAbsolutePosition(SubVI).vi"("Absolute Volume Position in Syringe (in ul)"=0.0 ("Volume to be Dispensed"), "Volume of Syringe"=w8757, "Resolution of Pumping"=w8755, "Flow Rate (ul/min)"=w8756, "VISA Refnum in"=w8758) -> ()  [unwired: 6 in, 1 out]
                            n8264 = local write "External Valve \nOpen"(TRUE ("External Valve \nOpen")) -> ()
                            n8265 = local write "Valve V5 Open"(FALSE ("Valve V5 Open")) -> ()
                            n8266 = local write "Valve V8 Open"(FALSE ("Valve V8 Open")) -> ()
                            n8267 = local write "Valve V6 Open"(FALSE ("Valve V6 Open")) -> ()
                            n8268 = local write "Valve V7 Open"(FALSE ("Valve V7 Open")) -> ()
                          }
                          frame #8 {
                            n8269 = local read "Initial Plunger Position"() -> (w8761:dbl)
                            n8270 = local read "Buffer-A2 Pumping\nResolution"() -> (w8760:T2)
                            n8271 = local read "VISA Refnum in\nfor Pump"() -> (w8762:refnum<visa-resource-name>)
                            n8272 = local read "Volume of Syringe"() -> (w8759:dbl)
                            n8273 = while {
                              tunnel: w8761 -> [w8768]
                              tunnel: w8762 -> [w8767]
                              tunnel: w8760 -> [w8766]
                              tunnel: w8759 -> [w8765]
                              stop <- w8763 stop-if-true
                              n8274 = Wait (ms)(milliseconds to wait=u32 100) -> ()  [unwired: 1 out]
                              n8275 = stacked-sequence {
                                tunnel: w8768 -> [w8774 _]
                                tunnel: w8767 -> [w8773 w8794]
                                tunnel: w8766 -> [w8772 _]
                                tunnel: w8765 -> [w8771 _]
                                tunnel: [_ w8791] -> w8763
                                frame #0 {
                                n8276 = call "AbsolutePlungerPosition (SubVI).vi"("VISA Refnum in"=w8773) -> ("Plunger Position"=w8770:i32)  [unwired: 10 in]
                                n8277 = case shown="\"Standard Pumping\", Default" w8772 {
                                tunnel: w8774 -> [w8779 w8788]
                                tunnel: w8770 -> [w8780 w8787]
                                tunnel: [w8778 w8785] -> w8769
                                tunnel: w8771 -> [w8777 w8786]
                                frame "Standard Pumping", Default {
                                n8278 = Subtract(x=w8779, y=w8780) -> (x-y=w8776:dbl)
                                n8279 = Absolute Value(x=w8776) -> (abs(x)=w8775:dbl)
                                n8280 = Multiply(x=w8775, y=w8777) -> (x*y=w8782:dbl)
                                n8281 = Divide(x=w8782, y=3000.0) -> (x/y=w8778:dbl)
                                }
                                frame "High Resolution Pumping" {
                                n8282 = Subtract(x=w8788, y=w8787) -> (x-y=w8784:dbl)
                                n8283 = Absolute Value(x=w8784) -> (abs(x)=w8783:dbl)
                                n8284 = Multiply(x=w8783, y=w8786) -> (x*y=w8790:dbl)
                                n8285 = Divide(x=w8790, y=24000.0) -> (x/y=w8785:dbl)
                                }
                                }
                                n8286 = local write "Volume being Injected \nin this process"(w8769) -> ()
                                }
                                frame #1 {
                                n8287 = local read "Stop for End of \nExperiment \nand Data Writing"() -> (w8793:bool)
                                n8288 = call "LSPOneStatus (SubVI).vi"("VISA Refnum in"=w8794) -> ("read buffer"=w8796:string)  [unwired: 10 in]
                                n8289 = call <vilib>:"Trim Whitespace.vi"("string"=w8796) -> ("trimmed string"=w8795:string)  [unwired: 1 in]
                                n8290 = Equal?(x=w8795, y="/0`\u0003") -> (x = y?=w8792:bool)
                                n8291 = Or(x=w8792, y=w8793) -> (x .or. y?=w8791:bool)
                                }
                              }
                            }
                          }
                          frame #9 {
                            n8292 = local read "Stop for End of \nExperiment \nand Data Writing"() -> (w8798:bool)
                            n8293 = local write "Pause Data Collection"(TRUE ("Pause Data Collection")) -> ()
                            n8294 = local write "Valve V3 Open"(FALSE ("Valve V3 Open")) -> ()
                            n8295 = local write "Valve V2 Open"(FALSE ("Valve V2 Open")) -> ()
                            n8296 = local write "Valve V4 Open"(FALSE ("Valve V4 Open")) -> ()
                            n8297 = local write "Start the Process"(FALSE) -> ()
                            n8298 = local write "Valve V1 Open"(FALSE ("Valve V1 Open")) -> ()
                            n8299 = case shown="True" w8798 {
                              frame False {
                              }
                              frame True {
                                n8300 = local read "VISA Refnum in\nfor Pump"() -> (w8809:refnum<visa-resource-name>)
                                n8301 = call "HardStopCurrentProcess (SubVI).vi"("VISA Refnum in"=w8809) -> ()  [unwired: 11 in]
                              }
                            }
                            n8302 = Wait (ms)(milliseconds to wait=u32 500) -> ()  [unwired: 1 out]
                            n8303 = local write "Valve V5 Open"(FALSE ("Valve V5 Open")) -> ()
                            n8304 = local write "Valve V6 Open"(FALSE ("Valve V6 Open")) -> ()
                            n8305 = local write "Valve V7 Open"(FALSE ("Valve V7 Open")) -> ()
                          }
                          frame #10 {
                            n8306 = local write "Volume being Injected \nin this process"(0.0 ("Volume being Injected \nin this process")) -> ()
                          }
                        }
                      }
                    }
                  }
                }
              }
              frame True {
                n8307 = local write "Pause Data Collection"(FALSE ("Pause Data Collection")) -> ()
              }
            }
          }
          frame "Single Column Wash Buffer-A" {
            n8308 = local read "Stopper that ends \nthe main loops"() -> (w8812:bool)
            n8309 = case shown="False" w8812 {
              frame False {
                n8310 = local read "Start the Process"() -> (w8813:bool)
                n8311 = case shown="True" w8813 {
                  frame False {
                    n8312 = local read "Stopper that ends \nthe main loops"() -> (w8815:bool)
                    n8313 = local read "Start the Process"() -> (w8814:bool)
                    n8314 = Or(x=w8815, y=w8814) -> (x .or. y?=w8816:bool)
                    n8315 = case shown="False" w8816 {
                      frame False {
                        n8316 = while {
                          stop <- w8819 stop-if-true
                          n8317 = local read "Stop for End of \nExperiment \nand Data Writing"() -> (w8818:bool)
                          n8318 = local read "Stopper that ends \nthe main loops"() -> (w8821:bool)
                          n8319 = local read "Start the Process"() -> (w8820:bool)
                          n8320 = Wait (ms)(milliseconds to wait=u32 10) -> ()  [unwired: 1 out]
                          n8321 = Or(x=w8821, y=w8820) -> (x .or. y?=w8819:bool)
                          n8322 = local write "Stopper that ends \nthe main loops"(w8818) -> ()
                        }
                        n8323 = One Button Dialog(message="Please Select the Process and Press 'Start the Process' Button") -> ()  [unwired: 1 in, 1 out]
                      }
                      frame True {
                      }
                    }
                  }
                  frame True {
                    n8324 = stacked-sequence {
                      frame #0 {
                        n8325 = local read "Buffer-A2 Volume \nto be Pumped"() -> (w8826:dbl)
                        n8326 = local read "Apparent Volume\nof Syringe"() -> (w8825:dbl)
                        n8327 = Quotient & Remainder(x=w8826, y=w8825) -> (x-y*floor(x/y)=w8823:dbl, floor(x/y)=w8824:dbl)
                        n8328 = for {
                          N: w8824 -> [_]
                          n8329 = stacked-sequence {
                            frame #0 {
                              # "Switch to Port-4"
                              # "Port-4 of pump is connected to Buffer-A"
                              n8330 = local read "VISA Refnum in\nfor Pump"() -> (w8828:refnum<visa-resource-name>)
                              n8331 = local read "Port for \nA2-Wash"() -> (w8827:string)
                              n8332 = call "PortChanger (SubVI).vi"("Port Number"=w8827, "VISA Refnum in"=w8828) -> ()  [unwired: 10 in]
                            }
                            frame #1 {
                              n8333 = local read "VISA Refnum in\nfor Pump"() -> (w8829:refnum<visa-resource-name>)
                              n8334 = call "ProcessCompletionWaiter (SubVI).vi"("VISA Refnum in"=w8829) -> ()  [unwired: 11 in]
                            }
                            frame #2 {
                              n8335 = local read "Buffer-A2 PickUp \nFlow Rate (ul/min)"() -> (w8832:dbl)
                              n8336 = local read "Buffer-A2 Pumping\nResolution"() -> (w8831:T2)
                              n8337 = local read "VISA Refnum in\nfor Pump"() -> (w8834:refnum<visa-resource-name>)
                              n8338 = local read "Apparent Volume\nof Syringe"() -> (w8830:dbl)
                              n8339 = local read "Volume of Syringe"() -> (w8833:dbl)
                              n8340 = call "RPickUp(SubVI).vi"("Volume to be picked up"=w8830, "Volume of Syringe"=w8833, "Resolution of PickUP"=w8831, "PickUp Flow Rate (ul/min)"=w8832, "VISA Refnum in"=w8834) -> ()  [unwired: 6 in, 1 out]
                            }
                            frame #3 {
                              n8341 = local read "Stopper that ends \nthe main loops"() -> (w8835:bool)
                              n8342 = local read "VISA Refnum in\nfor Pump"() -> (w8836:refnum<visa-resource-name>)
                              n8343 = case shown="True" w8835 {
                                frame False {
                                }
                                frame True {
                                n8344 = local read "VISA Refnum in\nfor Pump"() -> (w8837:refnum<visa-resource-name>)
                                n8345 = call "HardStopCurrentProcess (SubVI).vi"("VISA Refnum in"=w8837) -> ()  [unwired: 11 in]
                                }
                              }
                              n8346 = call "ProcessCompletionWaiter (SubVI).vi"("VISA Refnum in"=w8836) -> ()  [unwired: 11 in]
                            }
                            frame #4 {
                              # "Reads the initial Plunger Position for computing the volume dispensed"
                              n8347 = local read "VISA Refnum in\nfor Pump"() -> (w8839:refnum<visa-resource-name>)
                              n8348 = call "AbsolutePlungerPosition (SubVI).vi"("VISA Refnum in"=w8839) -> ("Plunger Position"=w8838:i32)  [unwired: 10 in]
                              n8349 = local write "Initial Plunger Position"(w8838) -> ()
                            }
                            frame #5 {
                              # "Switch to Port-2"
                              # "Port-2 of the pump is conncted to column-1 of chip"
                              n8350 = local read "VISA Refnum in\nfor Pump"() -> (w8841:refnum<visa-resource-name>)
                              n8351 = call "PortChanger (SubVI).vi"("Port Number"="2", "VISA Refnum in"=w8841) -> ()  [unwired: 10 in]
                            }
                            frame #6 {
                              n8352 = local read "Stopper that ends \nthe main loops"() -> (w8842:bool)
                              n8353 = local read "VISA Refnum in\nfor Pump"() -> (w8843:refnum<visa-resource-name>)
                              n8354 = case shown="True" w8842 {
                                frame False {
                                }
                                frame True {
                                n8355 = local read "VISA Refnum in\nfor Pump"() -> (w8844:refnum<visa-resource-name>)
                                n8356 = call "HardStopCurrentProcess (SubVI).vi"("VISA Refnum in"=w8844) -> ()  [unwired: 11 in]
                                }
                              }
                              n8357 = call "ProcessCompletionWaiter (SubVI).vi"("VISA Refnum in"=w8843) -> ()  [unwired: 11 in]
                            }
                            frame #7 {
                              # "Keeps the AMF valve after column-1 open and valve after column-2 closed"
                              n8358 = local read "Buffer-A2 Dispense\nFlow Rate (ul/min)"() -> (w8857:dbl)
                              n8359 = local read "Buffer-A2 Pumping\nResolution"() -> (w8856:T2)
                              n8360 = local read "VISA Refnum in\nfor Pump"() -> (w8859:refnum<visa-resource-name>)
                              n8361 = local write "Pause Data Collection"(FALSE ("Pause Data Collection")) -> ()
                              n8362 = local write "Valve V3 Open"(TRUE ("Valve V3 Open")) -> ()
                              n8363 = local write "Valve V4 Open"(TRUE ("Valve V4 Open")) -> ()
                              n8364 = local write "Valve V1 Open"(TRUE ("Valve V1 Open")) -> ()
                              n8365 = local write "Valve V2 Open"(FALSE ("Valve V2 Open")) -> ()
                              n8366 = local read "Volume of Syringe"() -> (w8858:dbl)
                              n8367 = call "GoToAbsolutePosition(SubVI).vi"("Absolute Volume Position in Syringe (in ul)"=0.0 ("Volume to be Dispensed"), "Volume of Syringe"=w8858, "Resolution of Pumping"=w8856, "Flow Rate (ul/min)"=w8857, "VISA Refnum in"=w8859) -> ()  [unwired: 6 in, 1 out]
                              n8368 = local write "External Valve \nOpen"(FALSE ("External Valve \nOpen")) -> ()
                              n8369 = local write "Valve V8 Open"(TRUE ("Valve V8 Open")) -> ()
                              n8370 = local write "Valve V5 Open"(TRUE ("Valve V5 Open")) -> ()
                              n8371 = local write "Valve V6 Open"(TRUE ("Valve V6 Open")) -> ()
                              n8372 = local write "Valve V7 Open"(TRUE ("Valve V7 Open")) -> ()
                            }
                            frame #8 {
                              n8373 = local read "Initial Plunger Position"() -> (w8862:dbl)
                              n8374 = local read "Buffer-A2 Pumping\nResolution"() -> (w8861:T2)
                              n8375 = local read "VISA Refnum in\nfor Pump"() -> (w8863:refnum<visa-resource-name>)
                              n8376 = local read "Volume of Syringe"() -> (w8860:dbl)
                              n8377 = while {
                                tunnel: w8862 -> [w8869]
                                tunnel: w8863 -> [w8868]
                                tunnel: w8861 -> [w8867]
                                tunnel: w8860 -> [w8866]
                                stop <- w8864 stop-if-true
                                n8378 = Wait (ms)(milliseconds to wait=u32 100) -> ()  [unwired: 1 out]
                                n8379 = stacked-sequence {
                                tunnel: w8869 -> [w8875 _]
                                tunnel: w8868 -> [w8874 w8895]
                                tunnel: w8867 -> [w8873 _]
                                tunnel: w8866 -> [w8872 _]
                                tunnel: [_ w8892] -> w8864
                                frame #0 {
                                n8380 = call "AbsolutePlungerPosition (SubVI).vi"("VISA Refnum in"=w8874) -> ("Plunger Position"=w8871:i32)  [unwired: 10 in]
                                n8381 = case shown="\"Standard Pumping\", Default" w8873 {
                                tunnel: w8875 -> [w8880 w8889]
                                tunnel: w8871 -> [w8881 w8888]
                                tunnel: [w8879 w8886] -> w8870
                                tunnel: w8872 -> [w8878 w8887]
                                frame "Standard Pumping", Default {
                                n8382 = Subtract(x=w8880, y=w8881) -> (x-y=w8877:dbl)
                                n8383 = Absolute Value(x=w8877) -> (abs(x)=w8876:dbl)
                                n8384 = Multiply(x=w8876, y=w8878) -> (x*y=w8883:dbl)
                                n8385 = Divide(x=w8883, y=3000.0) -> (x/y=w8879:dbl)
                                }
                                frame "High Resolution Pumping" {
                                n8386 = Subtract(x=w8889, y=w8888) -> (x-y=w8885:dbl)
                                n8387 = Absolute Value(x=w8885) -> (abs(x)=w8884:dbl)
                                n8388 = Multiply(x=w8884, y=w8887) -> (x*y=w8891:dbl)
                                n8389 = Divide(x=w8891, y=24000.0) -> (x/y=w8886:dbl)
                                }
                                }
                                n8390 = local write "Volume being Injected \nin this process"(w8870) -> ()
                                }
                                frame #1 {
                                n8391 = local read "Stop for End of \nExperiment \nand Data Writing"() -> (w8894:bool)
                                n8392 = call "LSPOneStatus (SubVI).vi"("VISA Refnum in"=w8895) -> ("read buffer"=w8897:string)  [unwired: 10 in]
                                n8393 = call <vilib>:"Trim Whitespace.vi"("string"=w8897) -> ("trimmed string"=w8896:string)  [unwired: 1 in]
                                n8394 = Equal?(x=w8896, y="/0`\u0003") -> (x = y?=w8893:bool)
                                n8395 = Or(x=w8893, y=w8894) -> (x .or. y?=w8892:bool)
                                }
                                }
                              }
                            }
                            frame #9 {
                              n8396 = local read "Stop for End of \nExperiment \nand Data Writing"() -> (w8899:bool)
                              n8397 = local write "Pause Data Collection"(TRUE ("Pause Data Collection")) -> ()
                              n8398 = local write "Valve V2 Open"(FALSE ("Valve V2 Open")) -> ()
                              n8399 = local write "Valve V1 Open"(FALSE ("Valve V1 Open")) -> ()
                              n8400 = Wait (ms)(milliseconds to wait=u32 500) -> ()  [unwired: 1 out]
                              n8401 = case shown="True" w8899 {
                                frame False {
                                }
                                frame True {
                                n8402 = local read "VISA Refnum in\nfor Pump"() -> (w8904:refnum<visa-resource-name>)
                                n8403 = call "HardStopCurrentProcess (SubVI).vi"("VISA Refnum in"=w8904) -> ()  [unwired: 11 in]
                                }
                              }
                            }
                            frame #10 {
                              n8404 = local write "Volume being Injected \nin this process"(0.0 ("Volume being Injected \nin this process")) -> ()
                            }
                          }
                        }
